vi "Agilent SNA Set Cal Off.vi"(6 "Channel":i8=1 min=1 max=99 step=1, 7 "Agilent SNA":T1, 8 "error in (no error)":errorcluster, 11 "VISA Resource Names":T2) -> (0 "error out":errorcluster {"code" format="%.0x"}, 3 "dup VISA Resource Names":T2)   [LabVIEW 2011]
doc: "This Vi for the HP8753B Network Analyzer is used to set averaging, smoothing, and the IF bandwidth."
uses:
  TypeDefs/Agilent SNA VISA.ctl
  TypeDefs/Agilent SNA Instrument Info.ctl
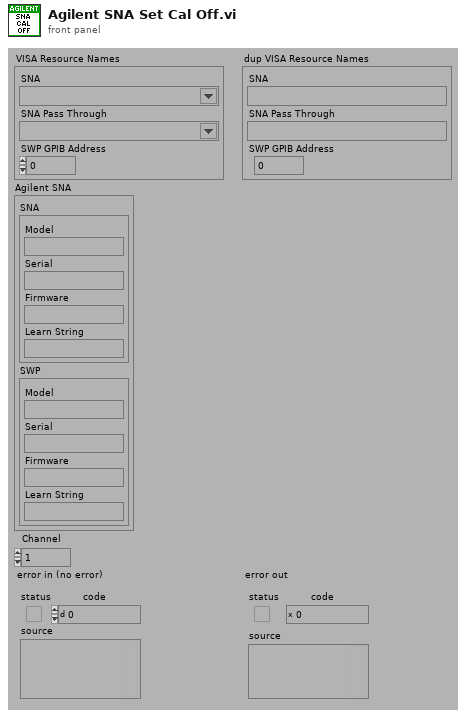
[diagram p1: front panel]
types:
  T1 = typedef "Agilent SNA Instrument Info.ctl" = cluster{"SNA":cluster{"Model":string, "Serial":string, "Firmware":string, "Learn String":string}, "SWP":cluster{"Model":string, "Serial":string, "Firmware":string, "Learn String":string}}
  T2 = typedef "Agilent SNA VISA.ctl" = cluster{"SNA":refnum<visa-resource-name>, "SNA Pass Through":refnum<visa-resource-name>, "SWP GPIB Address":i32}
  T3 = typedef "Agilent SNA Model.ctl" = enum16{"Not Supported", "8757X"}
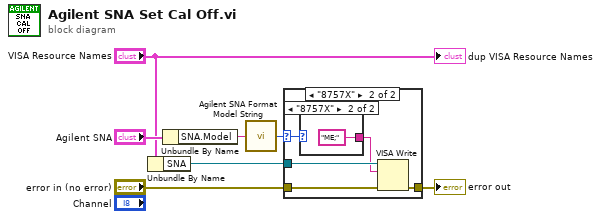
[diagram p0: block diagram]
diagram:
  n1 = Unbundle By Name("VISA Resource Names") -> ("SNA"=w2:refnum<visa-resource-name>)
  n2 = Unbundle By Name("Agilent SNA") -> ("SNA.Model"=w4:string)
  n3 = call "Agilent SNA Format Model String.vi"("Model String"=w4) -> ("Model"=w3:T3)
  n4 = case shown="\"8757X\"" w3 {
    selector: w3 -> [_ w9]
    tunnel: w2 -> [_ w13]
    tunnel: "error in (no error)" -> [w8 w12]
    tunnel: [w8 w11] -> w6
    frame "Not Supported" {
    }
    frame "8757X" {
      n5 = case shown="\"8757X\"" w9 {
        tunnel: [_ "ME;"] -> w10
        frame "Not Supported" {
        }
        frame "8757X" {
        }
      }
      n6 = VISA Write(VISA resource name=w13, write buffer=w10, error in (no error)=w12) -> (error out=w11:errorcluster)  [unwired: 2 out]
    }
  }
  "error out" <- w6
  "dup VISA Resource Names" <- "VISA Resource Names"
